vi "Closed-Loop.vi"(6 "Zero":dbl, 8 "Period":i64=500, 9 "Veloicty":dbl format="%.2f") -> (0 "error out":errorcluster, 2 "Voltage to Fans":dbl(graph), 3 "Velocity":dbl(graph))   [LabVIEW 2017]
uses:
  Globals/mainWTControl.vi
  <vilib>/addons/control/pid/pid.llb/PID Advanced (DBL).vi
  <vilib>/addons/control/pid/NI_PID_pid.lvlib
panel:
  in  "linearity":dbl=0.1 format="%.2f"
  in  "beta":dbl=1.0 format="%.2f"
  in  "auto? (T)":bool=TRUE
  in  "output range":cluster{"output high":dbl, "output low":dbl}={"output high"=6.0, "output low"=0.0} {"output low" format="%.2f"; "output high" format="%.2f"}
  in  "PID gains":T1={"proportional gain (Kc)"=0.05, "integral time (Ti, min)"=0.005, "derivative time (Td, min)"=0.0} {"derivative time (Td, min)" format="%.3f"; "integral time (Ti, min)" format="%.3f"; "proportional gain (Kc)" format="%.3f"}
  in  "setpoint range":cluster{"setpoint high":dbl, "setpoint low":dbl}={"setpoint high"=21.0, "setpoint low"=0.0} {"setpoint high" format="%.2f"; "setpoint low" format="%.2f"}
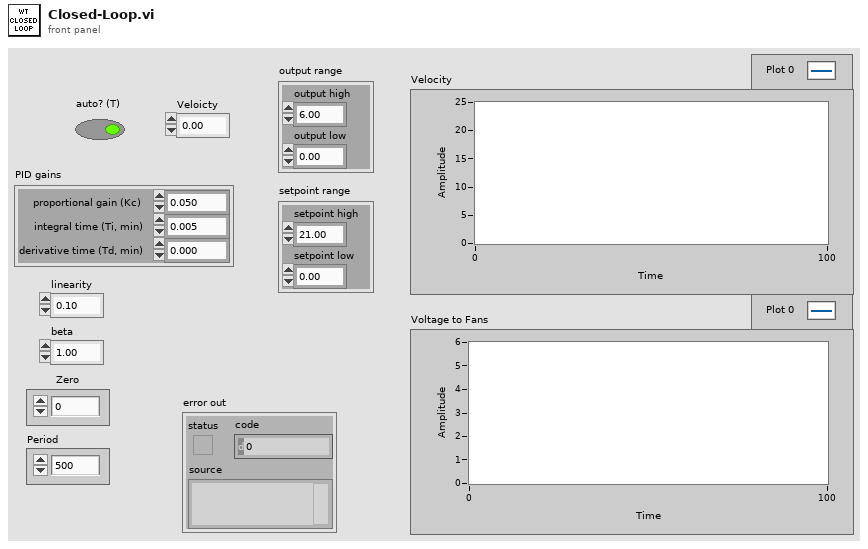
[diagram p1: front panel]
types:
  T1 = cluster{"proportional gain (Kc)":dbl, "integral time (Ti, min)":dbl, "derivative time (Td, min)":dbl}
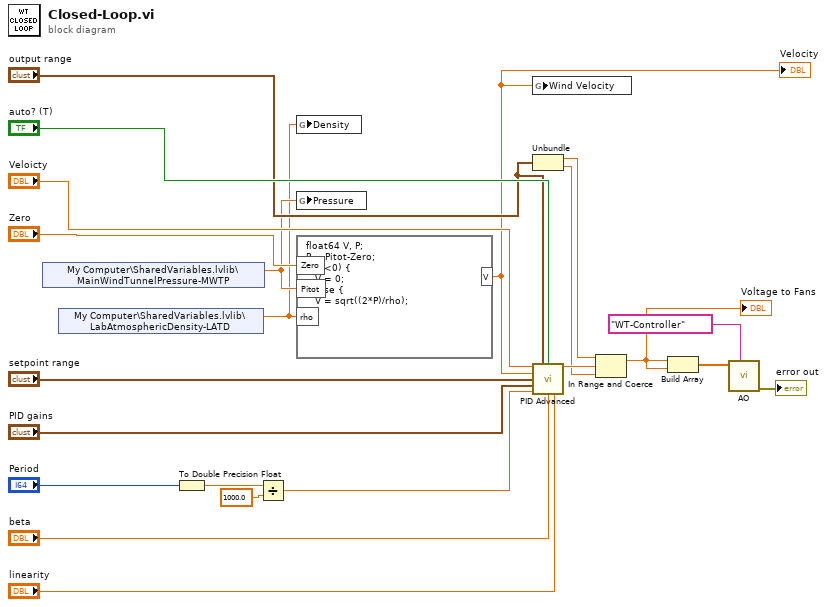
[diagram p0: block diagram]
diagram:
  n1 = shared-variable "My Computer\\SharedVariables.lvlib\\MainWindTunnelPressure-MWTP"() -> (w3:dbl)  [unwired: 1 in, 1 out]
  n2 = shared-variable "My Computer\\SharedVariables.lvlib\\LabAtmosphericDensity-LATD"() -> (w2:dbl)  [unwired: 1 in, 1 out]
  n3 = To Double Precision Float(number="Period") -> (double precision float=w18:dbl)
  n4 = Divide(x=w18, y=1000.0) -> (x/y=w9:dbl)
  n5 = global write "mainWTControl.vi" "Density"(w2) -> ()
  n6 = global write "mainWTControl.vi" "Pressure"(w3) -> ()
  n7 = formula code="float64 V, P;\nP = Pitot-Zero;\nif (P<0) {\n   V = 0;\n} else {\n   V = sqrt((2*P)/rho);\n}"("Zero"="Zero", "Pitot"=w3, "rho"=w2) -> ("V"=w4:dbl)
  "Velocity" <- w4
  n8 = global write "mainWTControl.vi" "Wind Velocity"(w4) -> ()
  n9 = Unbundle("output range") -> ("output high"=w6:dbl, "output low"=w5:dbl)
  n10 = call-poly <vilib>:"PID Advanced.vi"("setpoint"="Veloicty", "output range"="output range", "auto? (T)"="auto? (T)", "process variable"=w4, "setpoint range"="setpoint range", "PID gains"="PID gains", "dt (s)"=w9, "beta"="beta", "linearity"="linearity") -> ("output"=w12:dbl)  [unwired: 5 in, 1 out]
  n11 = In Range and Coerce(upper limit=w6, x=w12, lower limit=w5) -> (coerced(x)=w10:dbl)  [unwired: 1 out]
  "Voltage to Fans" <- w10
  n12 = Build Array(w10, w10) -> (w14:dbl[])
  n13 = call "AO.vi"("device name"=tag "WT-Controller", "data"=w14) -> ("error out"=→"error out":errorcluster)  [unwired: 5 in, 1 out]
